vi "DisplayAlertDialog.vi"(0 "reference in":refnum<class "LcWebView.lvclass">, 1 "Message":variant, 5 "Error In":errorcluster) -> (14 "reference out":refnum<class "LcWebView.lvclass">, 19 "Error Out":errorcluster)   [LabVIEW 2018, in "LcWebView.lvclass"]
uses:
  LcWebView.lvclass
  cdfa7b6c-348e-4618-b79e-b8b55caa0d01.vi
  <vilib>/JDP Science/JSONtext/Variant to JSON Text.vi
  <vilib>/JDP Science/JSONtext/LVClass Serializer/JSONtext LVClass Serializer.lvclass
panel:
  out "Result":string
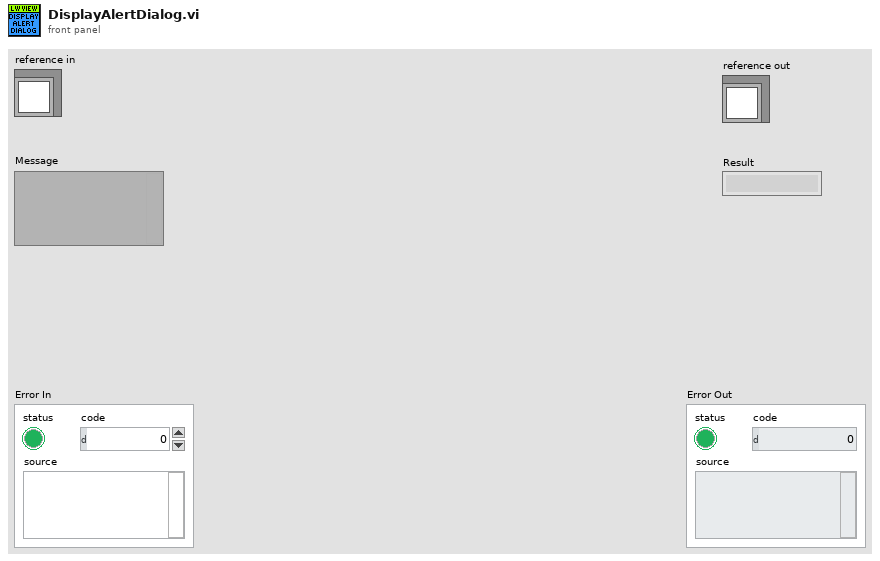
[diagram p1: front panel]
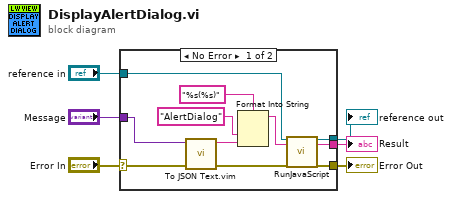
[diagram p0: block diagram]
diagram:
  n1 = case shown="No Error" "Error In" {
    selector: "Error In" -> [w9 w18]
    tunnel: [w10 w18] -> w3
    tunnel: [w11 w17] -> w4
    tunnel: "reference in" -> [w12 w17]
    tunnel: "Message" -> [w8 _]
    tunnel: [w7 _] -> w1
    frame No Error {
      n2 = call "To JSON Text.vim"("Anything"=w8) -> ("<JSON>"=w14:string)  [unwired: 9 in, 1 out]
      n3 = Format Into String(format string="%s(%s)", "AlertDialog" ("input 1"), w14) -> (resulting string=w13:string)  [unwired: 2 in, 1 out]
      n4 = call-dynamic "RunJavaScript.vi"("reference in"=w12, "Java Script Function"=w13, "Error In"=w9) -> ("reference out"=w11:refnum<class "LcWebView.lvclass">, "Result"=w7:string, "Error Out"=w10:errorcluster)  [unwired: 13 in, 1 out]
    }
    frame Error {
    }
  }
  "Error Out" <- w3
  "reference out" <- w4
  "Result" <- w1
